vi "robo_program.vi"(0 "VISA资源名称":refnum<visa-resource-name>, 1 "ax":i32, 2 "page":i32, 3 "file":string, 4 "错误输入（无错误）":errorcluster) -> (5 "VISA资源名称输出":refnum<visa-resource-name>, 6 "错误输出":errorcluster)   [LabVIEW 2017]
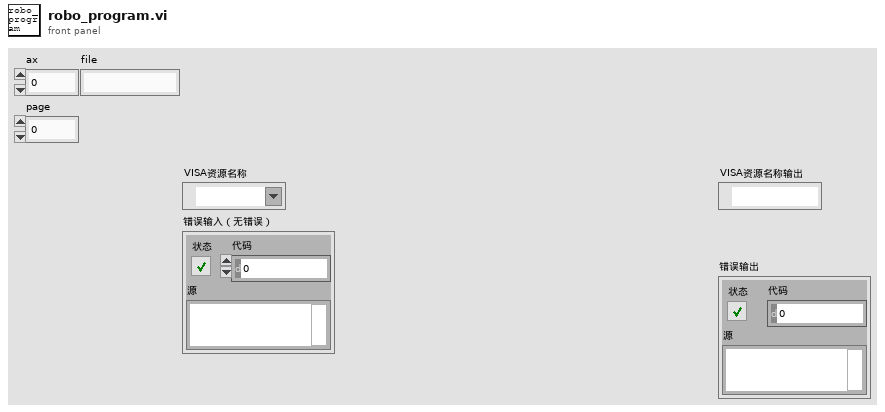
[diagram p1: front panel]
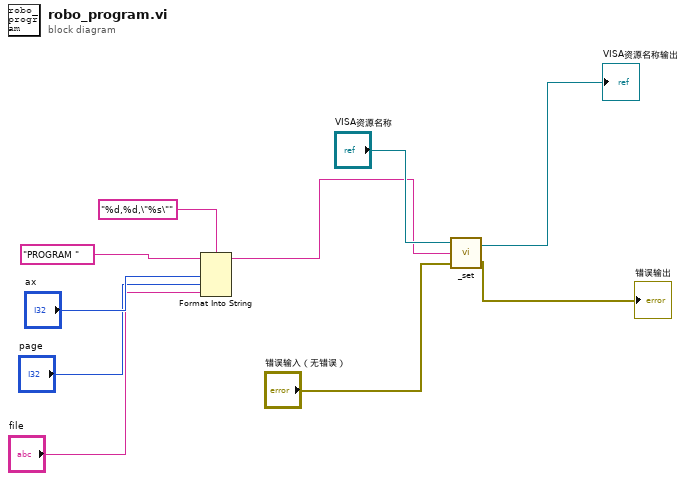
[diagram p0: block diagram]
diagram:
  n1 = Format Into String(format string="%d,%d,\"%s\"" ("格式字符串"), initial string="PROGRAM " ("初始字符串"), "ax", "page", "file") -> (resulting string=w4:string)  [unwired: 1 in, 1 out]
  n2 = call "_set.vi"("错误输入（无错误）"="错误输入（无错误）", "写入缓冲区"=w4, "连接ID"="VISA资源名称") -> ("错误输出"=→"错误输出":errorcluster, "连接ID输出"=→"VISA资源名称输出":refnum<k5>)
